vi "Determine If Belongs In Sector and Accumulate.vi"(6 "Left Sector Parameters":T2, 7 "Right Sector Parameters":T2, 8 "error in (no error)":errorcluster, 9 "Midpoint of Image":dbl, 10 "Starting Y Location":i32, 11 "Image Data":u8[][](array[numeric])) -> (0 "error out":errorcluster, 3 "[Accumulated Sectors]":T1[](array[typedef]))   [LabVIEW 2013]
uses:
  FPGA/Sector/Accumulate/Sector Parameter Cluster.ctl
  FPGA/Sector/Accumulate/Accumulated Sector Cluster.ctl
  FPGA/FPGA Image Processing.lvlib
panel:
  in  "Cancel Button":bool
  out "Progress":u16(slide) scale=0.0..1088.0
  # "Calculating Average Sector Background ..."
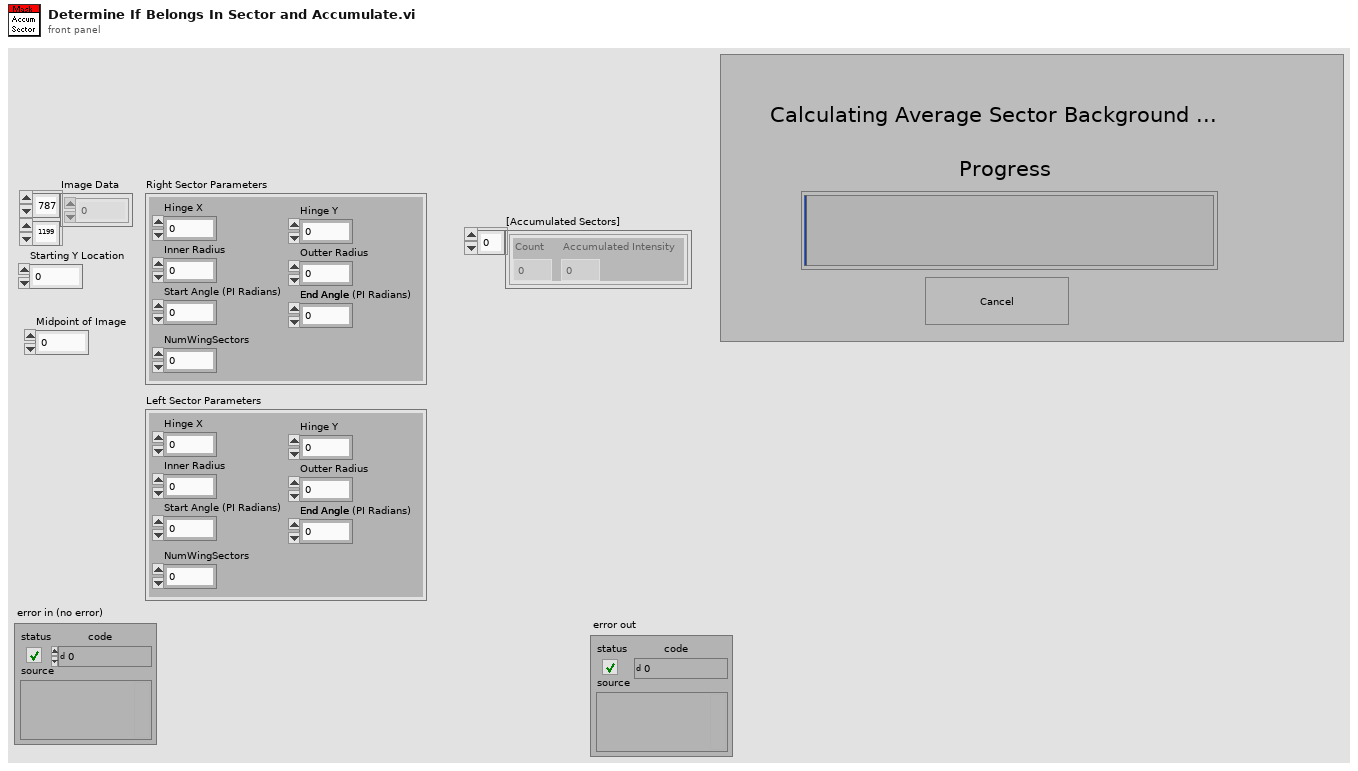
[diagram p1: front panel]
types:
  T1 = typedef "Accumulated Sector Cluster.ctl" = cluster{"Accumulated Intensity":u32, "Count":u16}
  T2 = typedef "Sector Parameter Cluster.ctl" = cluster{"Start Angle":fxp<+/-,17,2>, "End Angle":fxp<+,17,3>, "Inner Radius":u16, "Outter Radius":u16, "Hinge X":u16, "Hinge Y":u16, "NumWingSectors":u8}
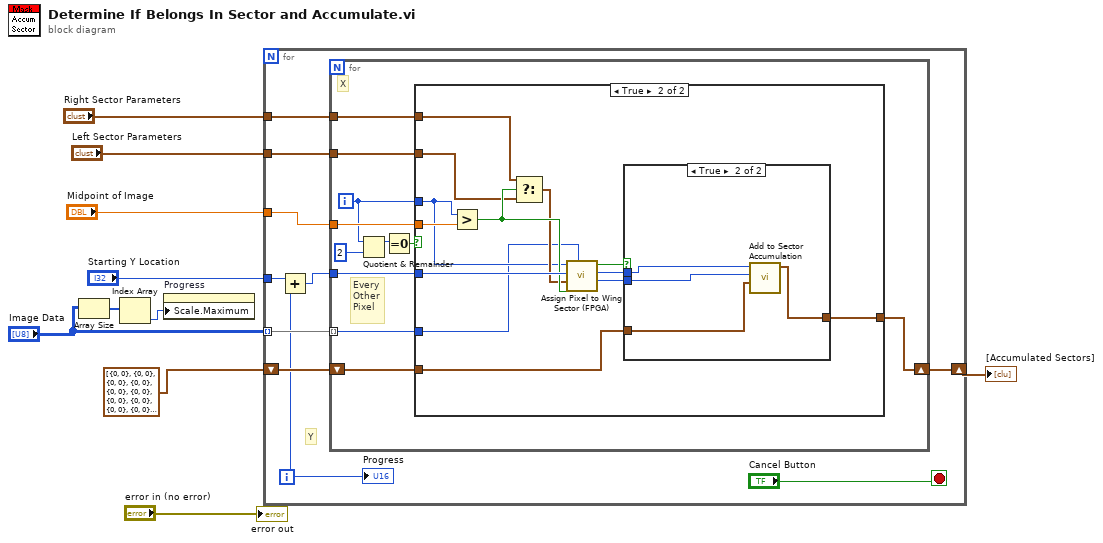
[diagram p0: block diagram]
diagram:
  n1 = Array Size(array="Image Data") -> (size(s)=w2:i32[])
  n2 = Index Array(array=w2) -> (element=w1:i32)  [unwired: 1 in]
  n3 = property on="Progress" class="Slide (strict)"("Scale.Maximum"=w1) -> ()  [unwired: 2 in, 2 out]
  n4 = for {
    tunnel: "Image Data" -> [w20] mode=indexing
    tunnel: "Midpoint of Image" -> [w19]
    tunnel: "Right Sector Parameters" -> [w18]
    tunnel: "Left Sector Parameters" -> [w17]
    shift-right: [w15] -> w5
    shift-left: T1[] [{"Accumulated Intensity"=0, "Count"=0}, {"Accumulated Intensity"=0, "Count"=0}, {"Accumulated Intensity"=0, "Count"=0}, {"Accumulated Intensity"=0, "Count"=0}, {"Accumulated Intensity"=0, "Count"=0}, {"Accumulated Intensity"=0, "Count"=0}, {"Accumulated Intensity"=0, "Count"=0}, {"Accumulated Intensity"=0, "Count"=0}, {"Accumulated Intensity"=0, "Count"=0}, {"Accumulated Intensity"=0, "Count"=0}, {"Accumulated Intensity"=0, "Count"=0}, {"Accumulated Intensity"=0, "Count"=0}, {"Accumulated Intensity"=0, "Count"=0}, {"Accumulated Intensity"=0, "Count"=0}, {"Accumulated Intensity"=0, "Count"=0}, {"Accumulated Intensity"=0, "Count"=0}, {"Accumulated Intensity"=0, "Count"=0}, {"Accumulated Intensity"=0, "Count"=0}, {"Accumulated Intensity"=0, "Count"=0}, {"Accumulated Intensity"=0, "Count"=0}, {"Accumulated Intensity"=0, "Count"=0}, {"Accumulated Intensity"=0, "Count"=0}, {"Accumulated Intensity"=0, "Count"=0}, {"Accumulated Intensity"=0, "Count"=0}, {"Accumulated Intensity"=0, "Count"=0}, {"Accumulated Intensity"=0, "Count"=0}, {"Accumulated Intensity"=0, "Count"=0}, {"Accumulated Intensity"=0, "Count"=0}, {"Accumulated Intensity"=0, "Count"=0}, {"Accumulated Intensity"=0, "Count"=0}, {"Accumulated Intensity"=0, "Count"=0}, {"Accumulated Intensity"=0, "Count"=0}] ("[Accumulated Sectors] Out") -> [w16]
    tunnel: "Starting Y Location" -> [w13]
    i -> [w12]
    stop <- "Cancel Button" stop-if-true
    # "Y"
    n5 = Add(x=w13, y=w12) -> (x+y=w14:i32)
    n6 = for {
      tunnel: w20 -> [w27] mode=indexing
      tunnel: w14 -> [w31]
      tunnel: w19 -> [w30]
      tunnel: w18 -> [w29]
      tunnel: w17 -> [w28]
      shift-right: [w25] -> w15
      shift-left: w16 -> [w26]
      i -> [w24]
      # "Every\nOther\nPixel"
      # "X"
      n7 = Quotient & Remainder(x=w24, y=2) -> (x-y*floor(x/y)=w22:i32)  [unwired: 1 out]
      n8 = Equal To 0?(x=w22) -> (x = 0?=w21:bool)
      n9 = case shown="True" w21 {
        tunnel: w31 -> [_ w45]
        tunnel: w30 -> [_ w44]
        tunnel: w29 -> [_ w42]
        tunnel: w28 -> [_ w41]
        tunnel: w24 -> [_ w39]
        tunnel: w27 -> [_ w38]
        tunnel: w26 -> [w32 w36]
        tunnel: [w32 w34] -> w25
        frame False {
        }
        frame True {
          n10 = Greater?(x=w39, y=w44) -> (0:w43:bool)
          n11 = Select(t=w42, s=w43, f=w41) -> (s? t:f=w40:T2)
          n12 = call "Assign Pixel to Wing Sector (FPGA).vi"("Pixel Intensity In"=w38, "Right Wing?"=w43, "Sector Parameters"=w40, "Pixel Y"=w45, "Pixel X"=w39) -> ("Pixel Intensity Out"=w33:u8, "sector #"=w35:u8, "output valid"=w37:bool)  [unwired: 1 in, 2 out]
          n13 = case shown="True" w37 {
            tunnel: w36 -> [w46 w48]
            tunnel: w35 -> [_ w50]
            tunnel: [w46 w47] -> w34
            tunnel: w33 -> [_ w49]
            frame False {
            }
            frame True {
              n14 = call "Add to Sector Accumulation.vi"("[Accumulated Sectors] In"=w48, "Pixel Intensity"=w49, "Sector ID"=w50) -> ("[Accumulated Sectors] Out"=w47:T1[])  [unwired: 8 in]
            }
          }
        }
      }
    }
    "Progress" <- w12
  }
  "[Accumulated Sectors]" <- w5
  "error out" <- "error in (no error)"
